vi "pareseXML_ChInfo.vi"(8 "error in (no error)":errorcluster, 11 "Raw Package without Header":string) -> (0 "error out":errorcluster, 3 "ChannelInfo":T1[](array[typedef]))   [LabVIEW 2020, in "OXYGEN_Datastream.lvlib"]
uses:
  OXYGEN_Datastream.lvlib
  TypeDefs/ChannelInfo.ctl
  TypeDefs/ChannelInfo_Scaling.ctl
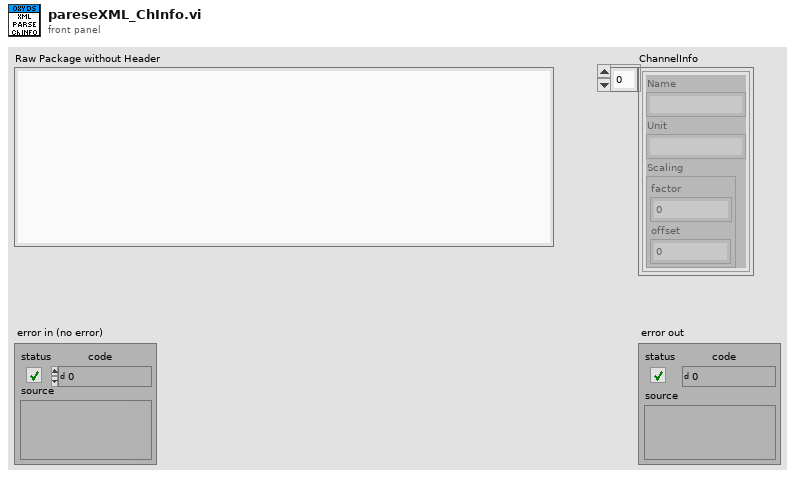
[diagram p1: front panel]
types:
  T1 = typedef "OXYGEN_Datastream.lvlib/ChannelInfo.ctl" = cluster{"Name":string, "Unit":string, "Scaling":T2}
  T2 = typedef "OXYGEN_Datastream.lvlib/ChannelInfo_Scaling.ctl" = cluster{"factor":dbl, "offset":dbl}
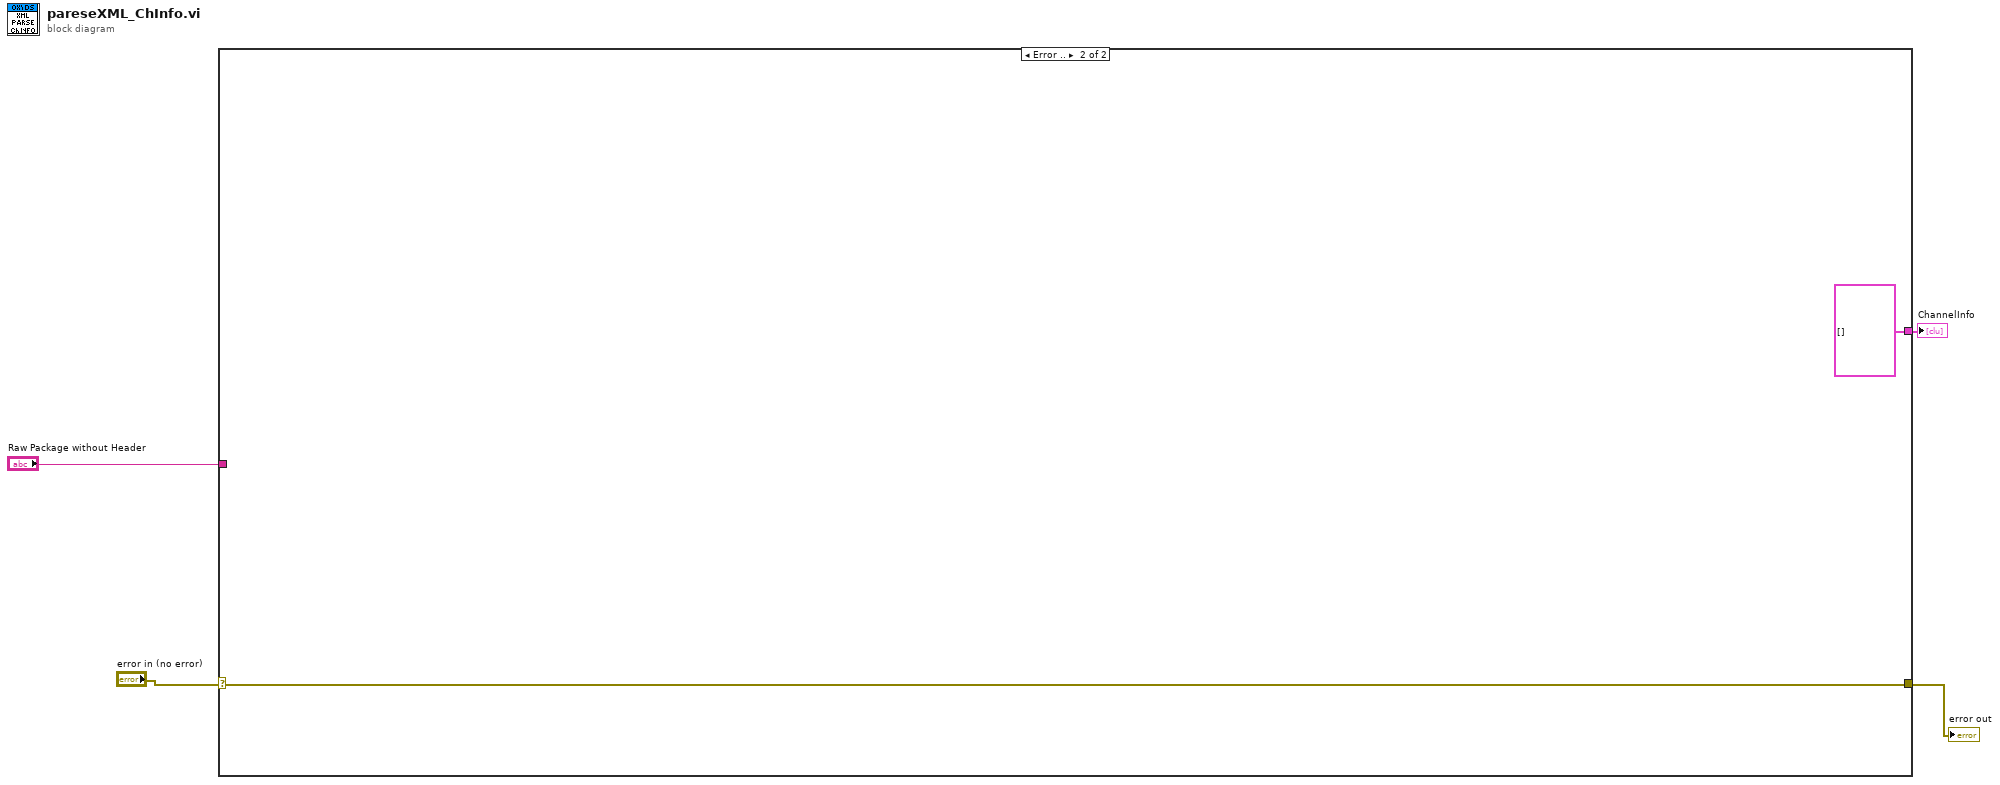
[diagram p0: block diagram]
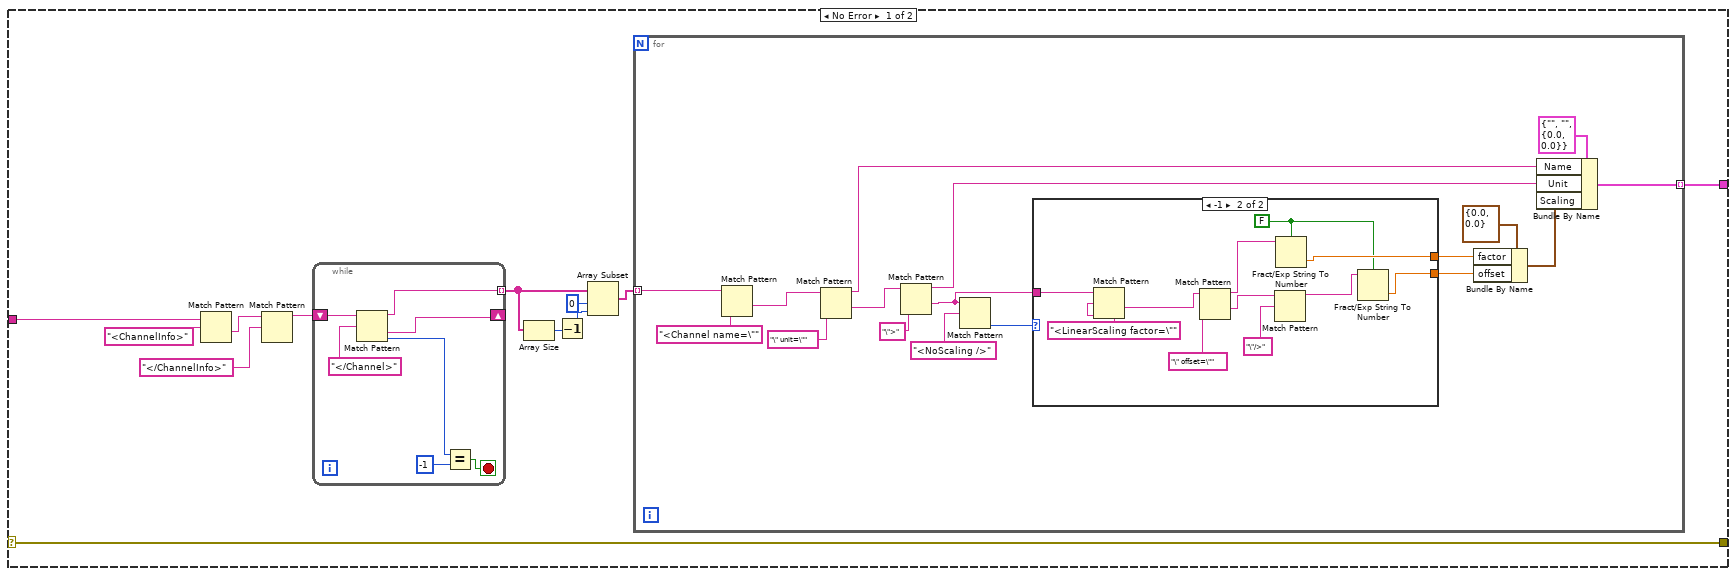
[diagram p2: hidden frame]
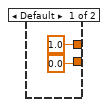
[diagram p3: hidden frame]
diagram:
  n1 = case shown="Error .." "error in (no error)" {
    selector: "error in (no error)" -> [w5 w54]
    tunnel: [w12 T1[] []] -> w4
    tunnel: "Raw Package without Header" -> [w6 _]
    tunnel: [w5 w54] -> w1
    frame No Error {
      n2 = Match Pattern(string=w6, regular expression="<ChannelInfo>") -> (after substring=w13:string)  [unwired: 1 in, 3 out]
      n3 = Match Pattern(string=w13, regular expression="</ChannelInfo>") -> (before substring=w16:string)  [unwired: 1 in, 3 out]
      n4 = while {
        shift-right: [w51] -> _
        shift-left: w16 -> [w53]
        tunnel: [w50] -> w9 mode=indexing
        stop <- w49 stop-if-true
        n5 = Match Pattern(string=w53, regular expression="</Channel>") -> (before substring=w50:string, after substring=w51:string, offset past match=w48:i32)  [unwired: 1 in, 1 out]
        n6 = Equal?(x=w48, y=-1) -> (x = y?=w49:bool)
      }
      n7 = Array Size(array=w9) -> (size(s)=w8:i32)
      n8 = Decrement(x=w8) -> (x-1=w7:i32)
      n9 = Array Subset(array=w9, index=0, length=w7) -> (w11:string[])
      n10 = for {
        tunnel: w11 -> [w33] mode=indexing
        tunnel: [w17] -> w12 mode=indexing
        n11 = Match Pattern(string=w33, regular expression="<Channel name=\"") -> (after substring=w31:string)  [unwired: 1 in, 3 out]
        n12 = Match Pattern(string=w31, regular expression="\" unit=\"") -> (before substring=w24:string, after substring=w29:string)  [unwired: 1 in, 2 out]
        n13 = Match Pattern(string=w29, regular expression="\">") -> (before substring=w23:string, after substring=w20:string)  [unwired: 1 in, 2 out]
        n14 = Match Pattern(string=w20, regular expression="<NoScaling />") -> (offset past match=w21:i32)  [unwired: 1 in, 3 out]
        n15 = case shown="-1" w21 {
          tunnel: w20 -> [_ w45]
          tunnel: [1.0 w40] -> w19
          tunnel: [0.0 w39] -> w18
          frame Default {
          }
          frame -1 {
            w36 = FALSE ("use system decimal point (T)")
            n16 = Match Pattern(string=w45, regular expression="<LinearScaling factor=\"") -> (after substring=w42:string)  [unwired: 1 in, 3 out]
            n17 = Match Pattern(string=w42, regular expression="\" offset=\"") -> (before substring=w37:string, after substring=w41:string)  [unwired: 1 in, 2 out]
            n18 = Match Pattern(string=w41, regular expression="\"/>") -> (before substring=w38:string)  [unwired: 1 in, 3 out]
            n19 = Fract/Exp String To Number(use system decimal point (T)=w36, string=w37) -> (number=w40:dbl)  [unwired: 2 in, 1 out]
            n20 = Fract/Exp String To Number(use system decimal point (T)=w36, string=w38) -> (number=w39:dbl)  [unwired: 2 in, 1 out]
          }
        }
        n21 = Bundle By Name(cluster=T2 {"factor"=0.0, "offset"=0.0} ("Scaling"), "factor"=w19, "offset"=w18) -> (w25:T2)
        n22 = Bundle By Name(cluster=T1 {"Name"="", "Unit"="", "Scaling"={"factor"=0.0, "offset"=0.0}} ("ChannelInfo"), "Name"=w24, "Unit"=w23, "Scaling"=w25) -> (w17:T1)
      }
    }
    frame Error {
    }
  }
  "ChannelInfo" <- w4
  "error out" <- w1
